vi "Thermometer.vi"() -> ()   [LabVIEW 2015]
uses:
  <vilib>/Utility/file.llb/Read From Spreadsheet File (DBL).vi
  <vilib>/Utility/file.llb/Read Delimited Spreadsheet (DBL).vi
  <vilib>/imath/engines/lvmath2/RunTimeEngine/Managers/WorkSpace/UID Generator.vi
  <vilib>/imath/engines/lvmath2/RunTimeEngine/ArithmeticOperatorToken/NIMS_ArithmeticOperator_rightdivmx.vi
  <instcachedir>/0/NIMS_ArithmeticOperator_rightdivmx_C61A2D056ED24171800131CCD8A24414.lvgen/NIMS_ArithmeticOperator_rightdivmx_C61A2D056ED24171800131CCD8A24414_003.vi
  <vilib>/imath/engines/lvmath2/RunTimeEngine/RunTimeType/NIMS_RunTimeType_From StrictType (excl LVString).vi
  <instcachedir>/0/NIMS_RunTimeType_From StrictType (excl LVString)_EB1C38A9BC5048DA9ABDA8F781E54D21.lvgen/NIMS_RunTimeType_From StrictType (excl LVString)_EB1C38A9BC5048DA9ABDA8F781E54D21_000.vi
  <vilib>/imathl/engines/lvmath/Functions/Error Handling/Create Error.vi
  <vilib>/imath/engines/lvmath2/RunTimeEngine/LocalVariableDefStatement/MC_LocalVariableDefStatement_Display.vi
  <vilib>/imath/engines/lvmath2/RunTimeEngine/IndexRead/NIMS V(S).vi
  <instcachedir>/0/NIMS V(S)_0488751826AF41519A22953C041130DC.lvgen/NIMS V(S)_0488751826AF41519A22953C041130DC_000.vi
  <vilib>/imath/engines/lvmath2/RunTimeEngine/ArithmeticOperatorToken/NIMS_ArithmeticOperator_powermx(M,M).vi
  <vilib>/imath/engines/lvmath2/RunTimeEngine/ArithmeticOperatorToken/NIMS_ArithmeticOperator_plus.vi
  <instcachedir>/0/NIMS_ArithmeticOperator_plus_A4F2756F5ADB4A0090E0DBD7C10701C8.lvgen/NIMS_ArithmeticOperator_plus_A4F2756F5ADB4A0090E0DBD7C10701C8_002.vi
  <vilib>/imath/engines/lvmath2/RunTimeEngine/ErrorHandling/NIMS_Create Error From Enums.vi
  <vilib>/imath/engines/lvmath/Functions/Error Handling/MergeErrorsWrapper.vi
  <vilib>/imath/engines/lvmath2/RunTimeEngine/ArithmeticOperatorToken/NIMS_ArithmeticOperator_rightdivmx(C,C).vi
  <instcachedir>/0/NIMS_ArithmeticOperator_rightdivmx(C,C)_8AB7F1F477EE4166BF59ADE0F95BCF66.lvgen/NIMS_ArithmeticOperator_rightdivmx(C,C)_8AB7F1F477EE4166BF59ADE0F95BCF66_000.vi
  <vilib>/imath/engines/lvmath2/RunTimeEngine/NodeEndStatement/NIMS_NodeEndStatement_Get Scalar.vi
  <instcachedir>/0/NIMS_NodeEndStatement_Get Scalar_EFB59FDA1E10412DB5B4364F310E1970.lvgen/NIMS_NodeEndStatement_Get Scalar_EFB59FDA1E10412DB5B4364F310E1970_000.vi
  <vilib>/imath/engines/lvmath2/RunTimeEngine/Managers/SymbolTable/Clear UID.vi
  <vilib>/imath/engines/lvmath2/RunTimeEngine/NodeEndStatement/NIMS_NodeEndStatement_Output.vi
  <instcachedir>/0/NIMS_NodeEndStatement_Output_53EC0D466D134D7ABD903AC30B43404B.lvgen/NIMS_NodeEndStatement_Output_53EC0D466D134D7ABD903AC30B43404B_001.vi
  <vilib>/imath/engines/lvmath2/RunTimeEngine/ErrorHandling/NIMS_Finalize Error.vi
  <vilib>/imath/engines/lvmath2/RunTimeEngine/Managers/SymbolTable/NIMS_WorkSpace.lvlib
panel:
  in  "Tab Control":enum32{"Beta", "Steinhart - Hart", "LSQ Fit"}(tab)
  out "Farenheit":dbl(slide) scale=0.0..100.0
  out "Celsius":dbl(slide) scale=0.0..100.0
  out "Kelvin":dbl(slide) scale=0.0..100.0 scale format="%#_6p"
  in  "Beta":dbl
  in  "R_0":dbl
  in  "T_0":dbl
  in  "Input measured voltage OR resistance of thermistor":enum32{"Voltage", "Resistance"}(tab)
  in  "Voltage In":dbl
  in  "Value of known resistor in voltage divider":dbl
  out "Voltage Out":dbl
  out "Thermistor Resistance":dbl
  in  "Resistance":dbl
  in  "Tab Control 2":enum32{"Constants from file", "Input"}(tab)
  in  "Steinhart-Hart Constants":path
  out "A 2":ext
  out "B 2":ext
  out "C 2":ext
  in  "C":dbl
  in  "B":dbl
  in  "A":dbl
  in  "Input measured voltage OR resistance of thermistor":enum32{"Voltage", "Resistance"}(tab)
  in  "Voltage In":dbl
  in  "Value of known resistor in voltage divider":dbl
  out "Voltage Out":dbl
  out "Thermistor Resistance":dbl
  in  "Resistance":dbl
  out "Farenheit":dbl(slide) scale=0.0..100.0
  out "Celsius":dbl(slide) scale=0.0..100.0
  out "Kelvin":dbl(slide) scale=0.0..100.0 scale format="%#_6p"
  in  "Coefficients Path":path
  out "Kelvin":dbl(slide) scale=0.0..100.0 scale format="%#_6p"
  out "Celsius":dbl(slide) scale=0.0..100.0
  out "Farenheit":dbl(slide) scale=0.0..100.0
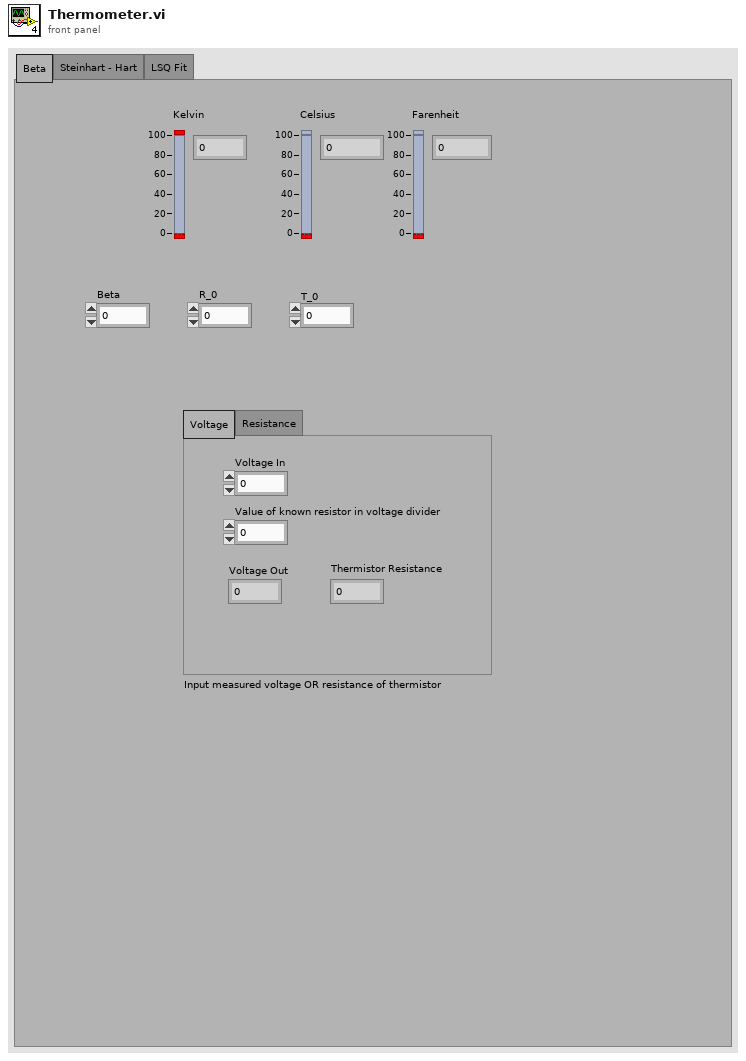
[diagram p1: front panel]
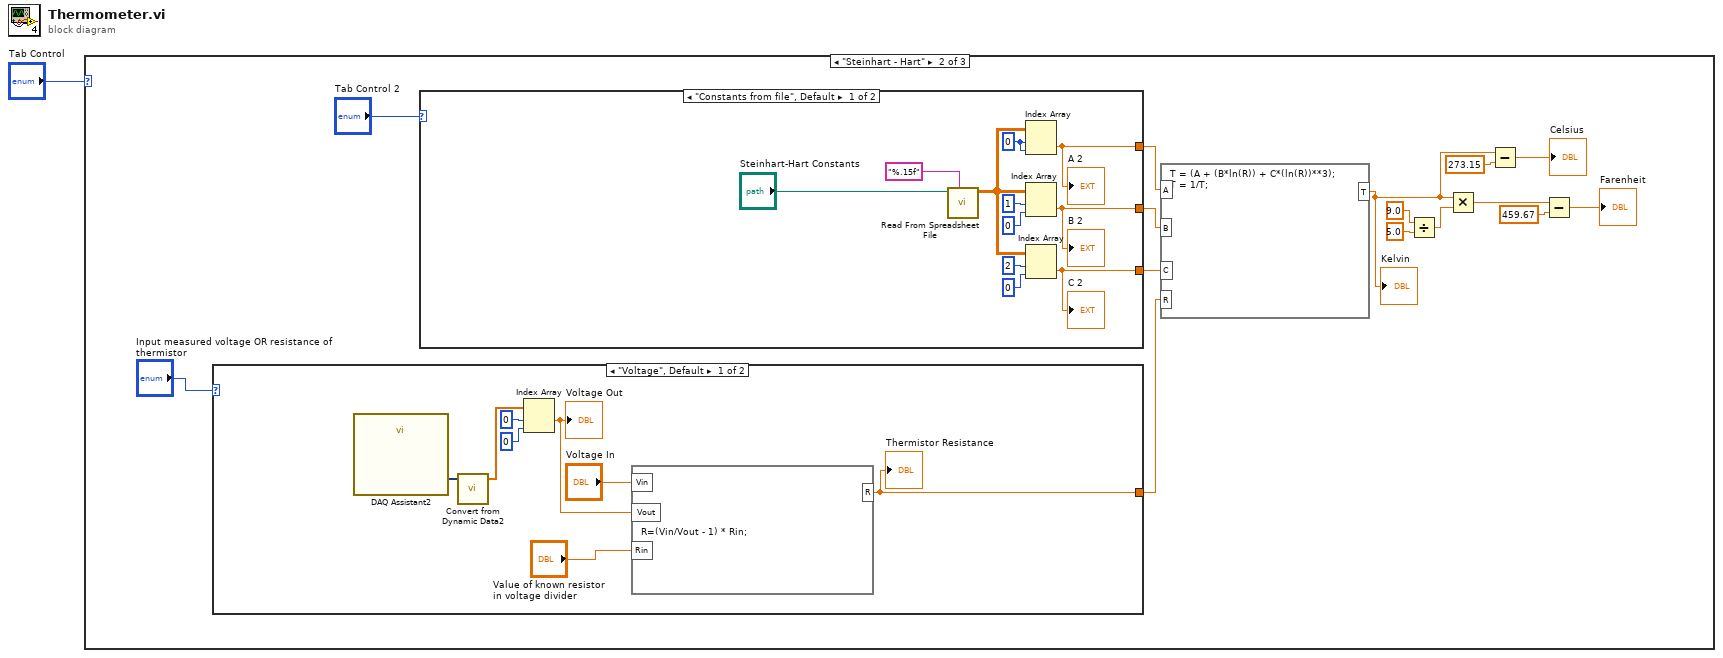
[diagram p0: block diagram]
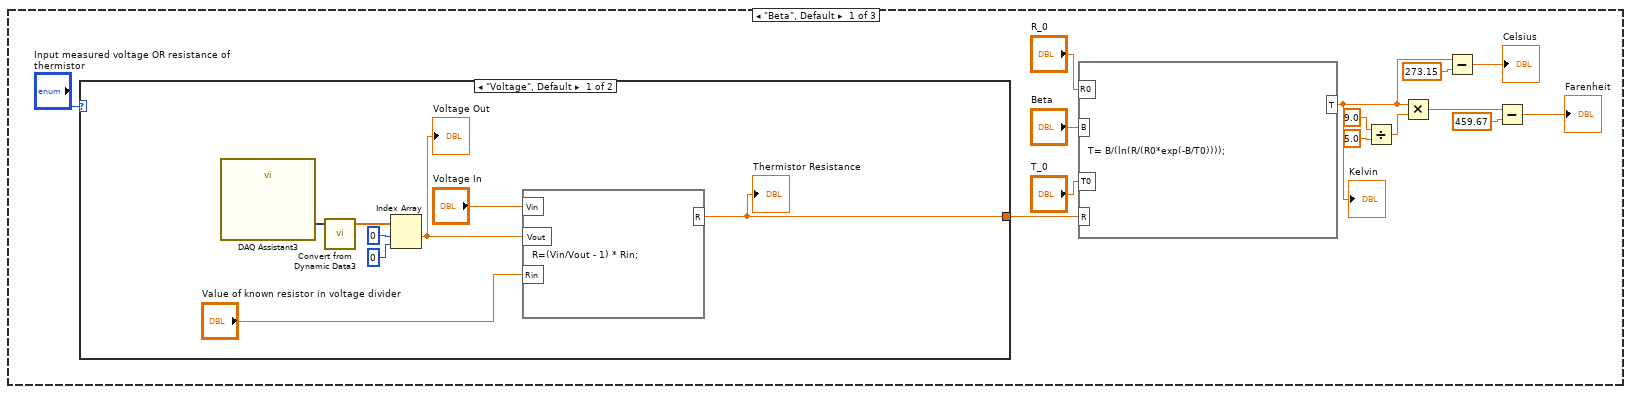
[diagram p2: hidden frame]
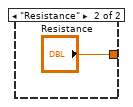
[diagram p3: hidden frame]
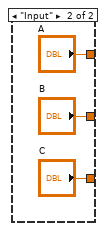
[diagram p4: hidden frame]
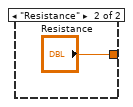
[diagram p5: hidden frame]
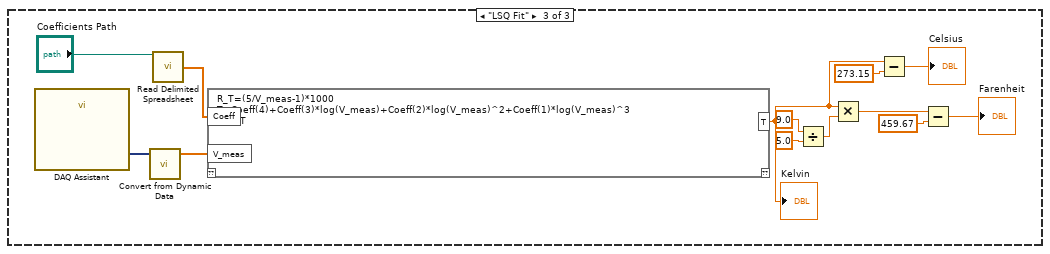
[diagram p6: hidden frame]
diagram:
  n1 = case shown="\"Steinhart - Hart\"" "Tab Control" {
    frame "Beta", Default {
      n2 = case shown="\"Voltage\", Default" "Input measured voltage OR resistance of thermistor" {
        tunnel: [w23 "Resistance"] -> w2
        frame "Voltage", Default {
          n3 = call "DAQ Assistant3"() -> ("data"=w20:dynamicdata)  [unwired: 17 in, 2 out]
          n4 = call "Convert from Dynamic Data3"("Dynamic Data Type"=w20) -> ("Array"=w17:dbl[])  [unwired: 3 in]
          n5 = Index Array(array=w17, index #1=0 ("index"), index #2=0 ("index")) -> (element #1=w16:dbl)  [unwired: 1 out]
          "Voltage Out" <- w16
          n6 = formula code="R=(Vin/Vout - 1) * Rin;"("Vin"="Voltage In", "Vout"=w16, "Rin"="Value of known resistor in voltage divider") -> ("R"=w23:dbl)
          "Thermistor Resistance" <- w23
        }
        frame "Resistance" {
        }
      }
      n7 = formula code="T= B/(ln(R/(R0*exp(-B/T0))));"("R0"="R_0", "B"="Beta", "T0"="T_0", "R"=w2) -> ("T"=w5:dbl)
      "Kelvin" <- w5
      n8 = Divide(x=9.0, y=5.0) -> (x/y=w9:dbl)
      n9 = Multiply(x=w5, y=w9) -> (x*y=w8:dbl)
      n10 = Subtract(x=w5, y=273.15) -> (x-y=→"Celsius":dbl)
      n11 = Subtract(x=w8, y=459.67) -> (x-y=→"Farenheit":dbl)
    }
    frame "Steinhart - Hart" {
      n12 = case shown="\"Voltage\", Default" "Input measured voltage OR resistance of thermistor" {
        tunnel: [w61 "Resistance"] -> w38
        frame "Voltage", Default {
          n13 = call "DAQ Assistant2"() -> ("data"=w58:dynamicdata)  [unwired: 17 in, 2 out]
          n14 = call "Convert from Dynamic Data2"("Dynamic Data Type"=w58) -> ("Array"=w55:dbl[])  [unwired: 3 in]
          n15 = Index Array(array=w55, index #1=0 ("index"), index #2=0 ("index")) -> (element #1=w54:dbl)  [unwired: 1 out]
          "Voltage Out" <- w54
          n16 = formula code="R=(Vin/Vout - 1) * Rin;"("Vin"="Voltage In", "Vout"=w54, "Rin"="Value of known resistor in voltage divider") -> ("R"=w61:dbl)
          "Thermistor Resistance" <- w61
        }
        frame "Resistance" {
        }
      }
      n17 = case shown="\"Constants from file\", Default" "Tab Control 2" {
        tunnel: [w42 "A"] -> w27
        tunnel: [w41 "B"] -> w26
        tunnel: [w40 "C"] -> w25
        frame "Constants from file", Default {
          w46 = 0 ("index (row)")
          n18 = call-poly <vilib>:"Read From Spreadsheet File.vi"("format (%.3f)"="%.15f", "file path (dialog if empty)"="Steinhart-Hart Constants") -> ("all rows"=w43:dbl[][])  [unwired: 5 in, 4 out]
          n19 = Index Array(array=w43, index (row)=w46, index (col)=w46) -> (element=w42:dbl)
          "A 2" <- w42
          n20 = Index Array(array=w43, index (row)=1, index (col)=0 ("disabled index (col)")) -> (element=w41:dbl)
          "B 2" <- w41
          n21 = Index Array(array=w43, index (row)=2, index (col)=0 ("disabled index (col)")) -> (element=w40:dbl)
          "C 2" <- w40
        }
        frame "Input" {
        }
      }
      n22 = formula code="T = (A + (B*ln(R)) + C*(ln(R))**3);\nT = 1/T;"("A"=w27, "B"=w26, "C"=w25, "R"=w38) -> ("T"=w32:dbl)
      "Kelvin" <- w32
      n23 = Divide(x=9.0, y=5.0) -> (x/y=w33:dbl)
      n24 = Multiply(x=w32, y=w33) -> (x*y=w31:dbl)
      n25 = Subtract(x=w32, y=273.15) -> (x-y=→"Celsius":dbl)
      n26 = Subtract(x=w31, y=459.67) -> (x-y=→"Farenheit":dbl)
    }
    frame "LSQ Fit" {
      n27 = call "DAQ Assistant"() -> ("data"=w65:dynamicdata)  [unwired: 17 in, 2 out]
      n28 = call "Convert from Dynamic Data"("Dynamic Data Type"=w65) -> ("Array"=w64:dbl[])  [unwired: 3 in]
      n29 = call-poly <vilib>:"Read Delimited Spreadsheet.vi"("file path (dialog if empty)"="Coefficients Path") -> ("first row"=w66:dbl[])  [unwired: 9 in, 5 out]
      n30 = mathscript code="R_T=(5/V_meas-1)*1000\nT=Coeff(4)+Coeff(3)*log(V_meas)+Coeff(2)*log(V_meas)^2+Coeff(1)*log(V_meas)^3\nT=1/T"("Coeff"=w66, "V_meas"=w64) -> ("T"=w63:dbl)  [unwired: 1 in, 1 out]
      "Kelvin" <- w63
      n31 = Divide(x=9.0, y=5.0) -> (x/y=w71:dbl)
      n32 = Multiply(x=w63, y=w71) -> (x*y=w70:dbl)
      n33 = Subtract(x=w63, y=273.15) -> (x-y=→"Celsius":dbl)
      n34 = Subtract(x=w70, y=459.67) -> (x-y=→"Farenheit":dbl)
    }
  }
